vi "GetCurrentValues.vi"(8 "error in (no error)":errorcluster, 9 "DataGroups ChannelStatus":T1[](array[typedef]), 10 "OpState":variant, 11 "History":variant) -> (0 "error out":errorcluster, 2 "current values":T3[](array[typedef]))   [LabVIEW 2017, in "McsaTestPanel.lvlib"]
uses:
  <vilib>/addons/InsightCM/Devices/Shared/Mcsa/McsaTestPanel/McsaTestPanel.lvlib
  <vilib>/addons/InsightCM/MessageBus/Base/controls/TestPanelCurrentValues.ctl
  <vilib>/addons/InsightCM/MessageBus/Base/controls/KeyValuePair.ctl
  <vilib>/addons/InsightCM/MessageBus/Base/controls/TestPanelCurrentValue.ctl
  <vilib>/addons/InsightCM/MessageBus/Base/controls/TestPanelValue.ctl
  <vilib>/addons/InsightCM/Devices/Shared/Mcsa/McsaTestPanel/controls/ChannelStatus.ctl
  <vilib>/addons/InsightCM/MessageBus/Base/controls/TestPanelTimeSeries.ctl
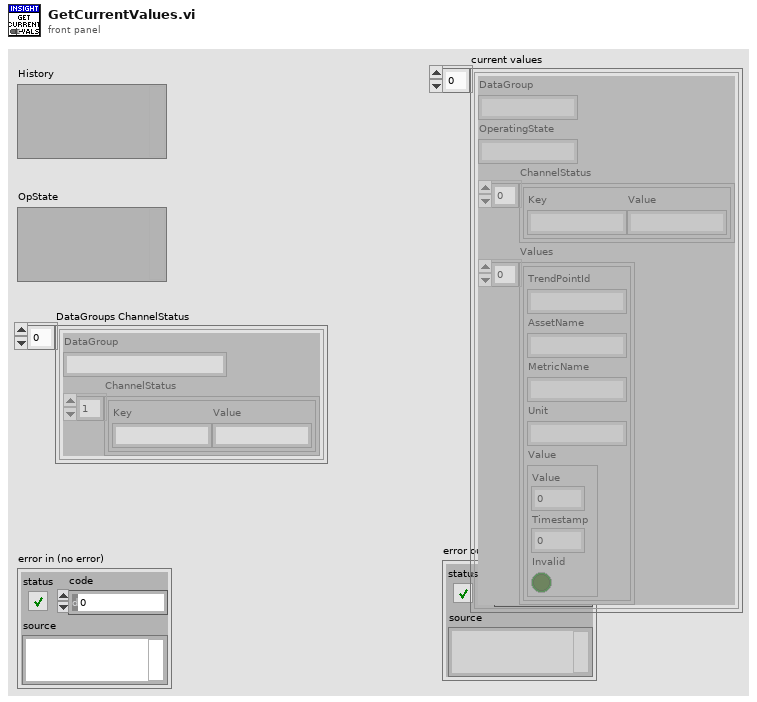
[diagram p1: front panel]
types:
  T1 = typedef "McsaTestPanel.lvlib/ChannelStatus.ctl" = cluster{"DataGroup":string, "ChannelStatus":T2[]}
  T2 = typedef "KeyValuePair.ctl" = cluster{"Key":string, "Value":string}
  T3 = typedef "TestPanelCurrentValues.ctl" = cluster{"DataGroup":string, "OperatingState":string, "ChannelStatus":T2[], "Values":T4[]}
  T4 = typedef "TestPanelCurrentValue.ctl" = cluster{"TrendPointId":string, "AssetName":string, "MetricName":string, "Unit":string, "Value":T5}
  T5 = typedef "TestPanelValue.ctl" = cluster{"Value":dbl, "Timestamp":i64, "Invalid":bool}
  T6 = typedef "TestPanelTimeSeries.ctl" = cluster{"TrendPointId":string, "AssetName":string, "MetricName":string, "Unit":string, "Values":T5[]}
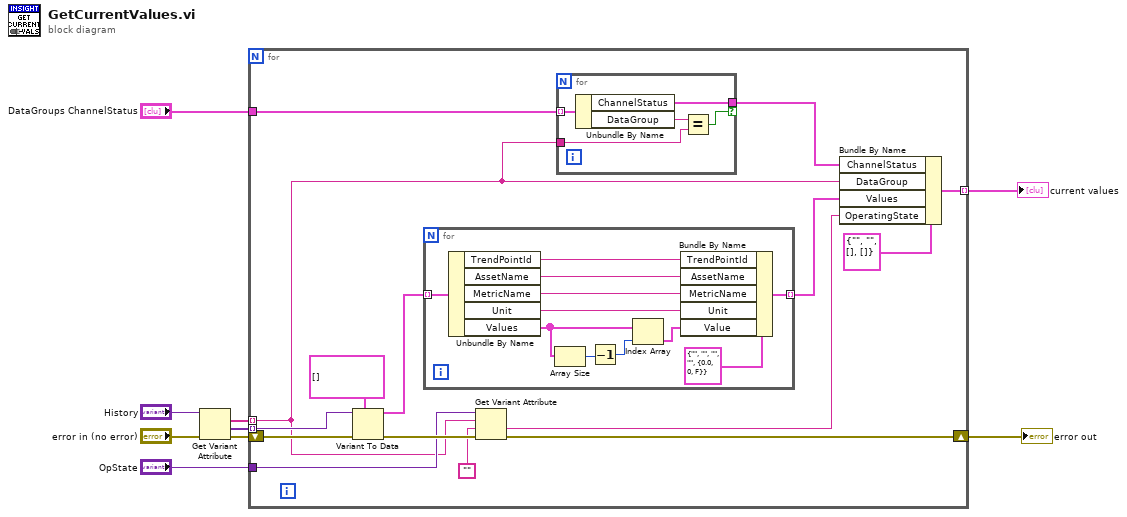
[diagram p0: block diagram]
diagram:
  n1 = Get Variant Attribute(Variant="History", error in="error in (no error)") -> (names=w6:string[], values=w7:variant[], error out=w8:errorcluster)  [unwired: 2 in, 1 out]
  n2 = for {
    shift-right: [w14] -> w3
    shift-left: w8 -> [w23]
    tunnel: w7 -> [w22] mode=indexing
    tunnel: w6 -> [w11] mode=indexing
    tunnel: "OpState" -> [w17]
    tunnel: [w13] -> w2 mode=indexing
    tunnel: "DataGroups ChannelStatus" -> [w12]
    n3 = Variant To Data(error in=w23, type=T6[] [], Variant=w22) -> (data=w20:T6[], error out=w18:errorcluster)
    n4 = for {
      tunnel: w20 -> [w31] mode=indexing
      tunnel: [w30] -> w19 mode=indexing
      n5 = Unbundle By Name(w31) -> ("TrendPointId"=w34:string, "AssetName"=w35:string, "MetricName"=w33:string, "Unit"=w32:string, "Values"=w39:T5[])
      n6 = Array Size(array=w39) -> (size(s)=w38:i32)
      n7 = Decrement(x=w38) -> (x-1=w37:i32)
      n8 = Index Array(array=w39, index=w37) -> (element=w36:T5)
      n9 = Bundle By Name(cluster=T4 {"TrendPointId"="", "AssetName"="", "MetricName"="", "Unit"="", "Value"={"Value"=0.0, "Timestamp"=0, "Invalid"=FALSE}} ("CurrentValue"), "TrendPointId"=w34, "AssetName"=w35, "MetricName"=w33, "Unit"=w32, "Value"=w36) -> (w30:T4)
    }
    n10 = Get Variant Attribute(Variant=w17, name=w11, default value (empty Variant)="", error in=w18) -> (value=w15:string, error out=w14:errorcluster)  [unwired: 2 out]
    n11 = for {
      tunnel: w12 -> [w29] mode=indexing
      tunnel: w11 -> [w27]
      tunnel: [w26] -> w10 if=w25
      n12 = Unbundle By Name(w29) -> ("ChannelStatus"=w26:T2[], "DataGroup"=w28:string)
      n13 = Equal?(x=w28, y=w27) -> (x = y?=w25:bool)
    }
    n14 = Bundle By Name(cluster=T3 {"DataGroup"="", "OperatingState"="", "ChannelStatus"=[], "Values"=[]} ("CurrentValues"), "ChannelStatus"=w10, "DataGroup"=w11, "Values"=w19, "OperatingState"=w15) -> (w13:T3)
  }
  "error out" <- w3
  "current values" <- w2
